vi "Parser_0xE1_(SubVI).vi"(11 "String in":string) -> (2 "Значение параметра":sgl, 3 "Номер параметра":i32)   [LabVIEW 2017, in "LV_Unicorn.lvlib"]
uses:
  LV_Unicorn.lvlib
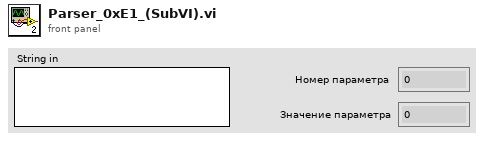
[diagram p1: front panel]
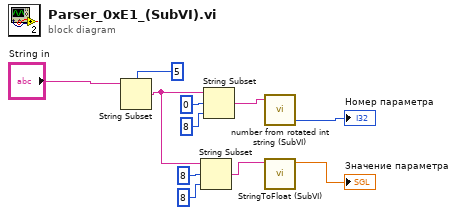
[diagram p0: block diagram]
diagram:
  n1 = String Subset(string="String in", offset (0)=5) -> (substring=w3:string)  [unwired: 1 in]
  n2 = String Subset(string=w3, offset (0)=8, length (rest)=8 ("length (rest)")) -> (substring=w2:string)
  n3 = String Subset(string=w3, offset (0)=0, length (rest)=8 ("length (rest)")) -> (substring=w9:string)
  n4 = call "number from rotated int string (SubVI).vi"("String"=w9) -> ("int number"=→"Номер параметра":i32)  [unwired: 2 in, 2 out]
  n5 = call "StringToFloat (SubVI).vi"("String in"=w2) -> ("Numeric"=→"Значение параметра":sgl)  [unwired: 10 in]
